vi "Balancing Controller.vi"(6 "Configuration":T1={"Accelerometer Bias"={"X (m/s)"=0.0, "Y (m/s)"=0.0, "Z (m/s)"=0.0}, "Gyroscope Bias"={"X (m/s)"=0.0, "Y (m/s)"=0.0, "Z (m/s)"=0.0}, "Steering Motor Gear Ratio"=611.0, "Steering Pully Gear Ratio"=1.0, "Steering Encoder CPR"=500.0, "Steering Motor Max RPM"=4000.0, "Wheelbase (m)"=1.12, "Fork Angle (rad)"=1.3, "Balancing Controller"={"Kp (/s)"=0.05, "Kd (1)"=0.0}, "Max Allowed Steering Angle (rad)"=0.7, "Task Periods"={"Emergency Stop (us)"=0, "IMU (us)"=0, "Steering Motor Encoder (us)"=0, "State Estimator (us)"=0, "Balancing Controller (us)"=0, "GNSS (us)"=0}}, 8 "Measurement In":refnum<data-value>, 9 "State Estimate In":refnum<data-value>, 11 "Error In":errorcluster) -> (0 "Measurement Out":refnum<data-value>, 1 "State Estimate Out":refnum<data-value>, 3 "Error Out":errorcluster, 4 "Steering Angle Rate (rad/s)":dbl)   [LabVIEW 2019]
uses:
  State Estimator/State Estimate.ctl
  Configuration/Configuration.ctl
  State Estimator/Measurements.ctl
  IMU/IMU Data.ctl
  Steering Motor Encoder/Steering Motor Encoder Data.ctl
  GNSS/GNSS Data.ctl
  Logging/Log Level.ctl
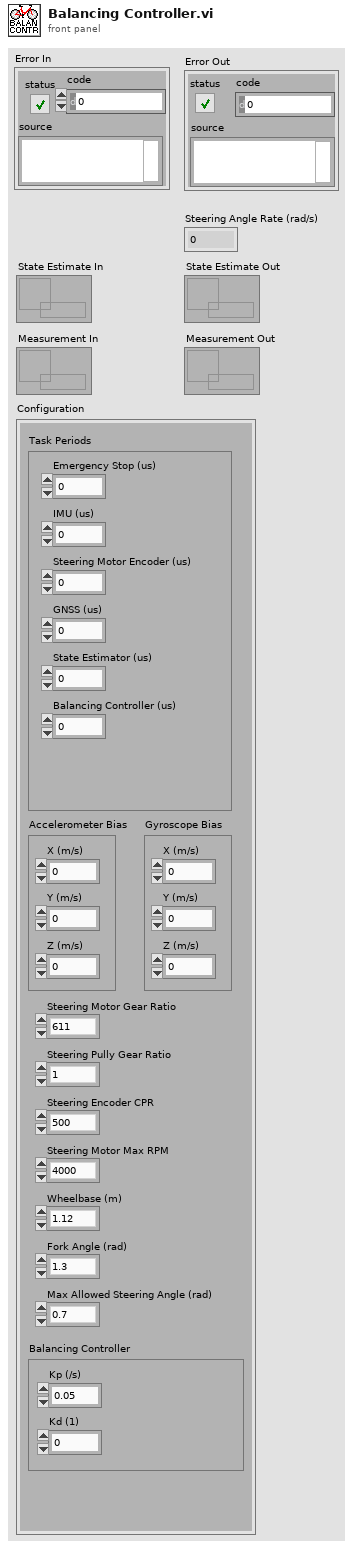
[diagram p1: front panel]
types:
  T1 = typedef "Configuration.ctl" = cluster{"Accelerometer Bias":cluster{"X (m/s)":dbl, "Y (m/s)":dbl, "Z (m/s)":dbl}, "Gyroscope Bias":cluster{"X (m/s)":dbl, "Y (m/s)":dbl, "Z (m/s)":dbl}, "Steering Motor Gear Ratio":dbl, "Steering Pully Gear Ratio":dbl, "Steering Encoder CPR":dbl, "Steering Motor Max RPM":dbl, "Wheelbase (m)":dbl, "Fork Angle (rad)":dbl, "Balancing Controller":cluster{"Kp (/s)":dbl, "Kd (1)":dbl}, "Max Allowed Steering Angle (rad)":dbl, "Task Periods":cluster{"Emergency Stop (us)":i64, "IMU (us)":i64, "Steering Motor Encoder (us)":i64, "State Estimator (us)":i64, "Balancing Controller (us)":i64, "GNSS (us)":i64}}
  T2 = typedef "Log Level.ctl" = enum16{"Error", "Warning", "Info"}
  T3 = typedef "Measurements.ctl" = cluster{"IMU Data":T4, "Steering Motor Encoder Data":T5, "GNSS Data":T6}
  T4 = typedef "IMU Data.ctl" = cluster{"Gyroscope":cluster{"X (rad/s)":dbl, "Y (rad/s)":dbl, "Z (rad/s)":dbl}, "Accelerometer":cluster{"X (m/s^2)":dbl, "Y (m/s^2)":dbl, "Z (m/s^2)":dbl}}
  T5 = typedef "Steering Motor Encoder Data.ctl" = cluster{"Encoder Position (counts)":i32, "Steering Angle (rad)":dbl}
  T6 = typedef "GNSS Data.ctl" = cluster{"Latitude (rad)":dbl, "Longitude (rad)":dbl, "Altitude (m)":dbl, "Speed (m/s)":dbl, "Heading (rad)":dbl, "Fix Quality":i32, "Number of Satellites":i32, "Latitude (deg)":dbl, "Longitude (deg)":dbl}
  T7 = typedef "State Estimate.ctl" = cluster{"X (m)":dbl, "Y (m)":dbl, "Psi (rad)":dbl, "Roll (rad)":dbl, "Roll Rate (rad/s)":dbl}
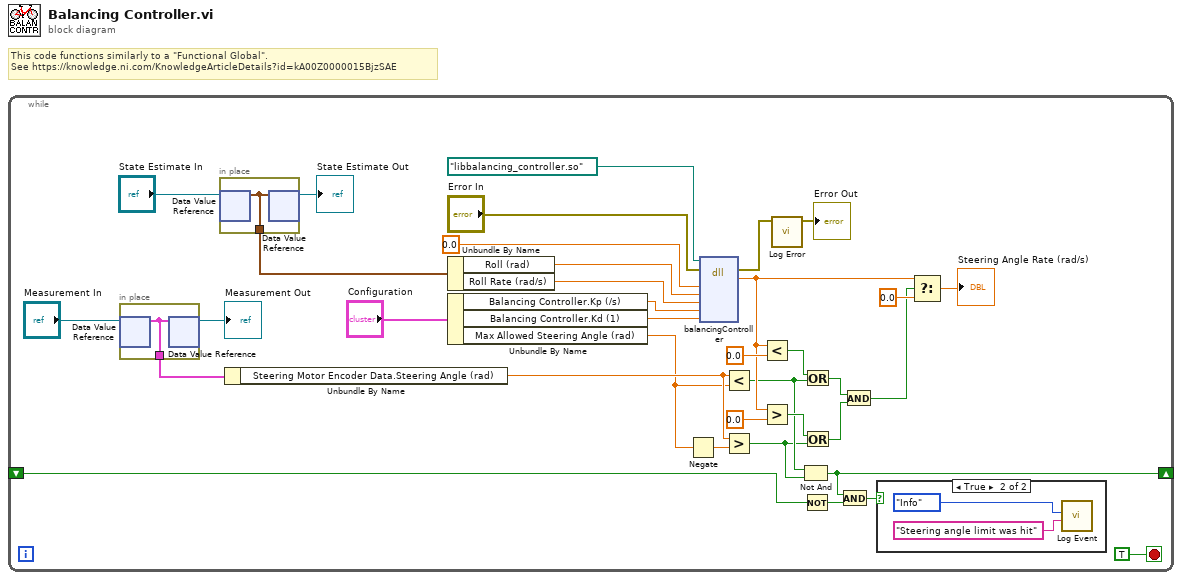
[diagram p0: block diagram]
diagram:
  # "This code functions similarly to a \"Functional Global\".\nSee https://knowledge.ni.com/KnowledgeArticleDetails?id=kA00Z0000015BjzSAE"
  n1 = while {
    shift-right: [w3] -> _
    shift-left: _ -> [w5]
    stop <- TRUE stop-if-true
    n2 = in-place {
      in-place-border: [w39] -> w23
      n3 = in-place-dvr #1("Measurement In") -> (w39:T3)  [unwired: 1 out]
      n4 = in-place-dvr #1(w39) -> (→"Measurement Out":refnum<data-value>)  [unwired: 1 out]
    }
    n5 = in-place {
      in-place-border: [w40] -> w26
      n6 = in-place-dvr #2("State Estimate In") -> (w40:T7)  [unwired: 1 out]
      n7 = in-place-dvr #2(w40) -> (→"State Estimate Out":refnum<data-value>)  [unwired: 1 out]
    }
    n8 = Unbundle By Name(w23) -> ("Steering Motor Encoder Data.Steering Angle (rad)"=w11:dbl)
    n9 = Unbundle By Name(w26) -> ("Roll (rad)"=w32:dbl, "Roll Rate (rad/s)"=w31:dbl)
    n10 = Unbundle By Name("Configuration") -> ("Balancing Controller.Kp (/s)"=w29:dbl, "Balancing Controller.Kd (1)"=w28:dbl, "Max Allowed Steering Angle (rad)"=w10:dbl)
    n11 = Negate(x=w10) -> (-x=w12:dbl)
    n12 = dll-call lib="?" fn="balancingController"(path in=path "libbalancing_controller.so", error in="Error In", "rollReference"=0.0, "roll"=w32, "rollRate"=w31, "Kp"=w29, "Kd"=w28) -> (error out=w8:errorcluster, "Steering Angle Rate"=w16:dbl)  [unwired: 6 in, 1 out]
    n13 = Less?(x=w11, y=w10) -> (x < y?=w2:bool)
    n14 = Greater?(x=w11, y=w12) -> (0:w1:bool)
    n15 = Less?(x=w16, y=0.0) -> (x < y?=w19:bool)
    n16 = Greater?(x=w16, y=0.0) -> (0:w15:bool)
    n17 = call "Log Error.vi"("Error In"=w8) -> ("Error Out"=→"Error Out":errorcluster)  [unwired: 10 in]
    n18 = Not And(1:w1, 2:w2) -> (0:w3:bool)
    n19 = Not(x=w5) -> (.not. x?=w6:bool)
    n20 = Or(x=w19, y=w2) -> (x .or. y?=w18:bool)
    n21 = Or(x=w15, y=w1) -> (x .or. y?=w14:bool)
    n22 = And(x=w3, y=w6) -> (x .and. y?=w4:bool)
    n23 = And(x=w18, y=w14) -> (x .and. y?=w13:bool)
    n24 = case shown="True" w4 {
      frame False {
      }
      frame True {
        n25 = call "Log Event.vi"("Message"="Steering angle limit was hit", "Log Level"=Log_Level."Info") -> ()  [unwired: 9 in, 1 out]
      }
    }
    n26 = Select(t=w16, s=w13, f=0.0) -> (s? t:f=→"Steering Angle Rate (rad/s)":dbl)
  }
